vi "ExpandSearch.vi"(8 "error in (no error)":errorcluster, 11 "Waypoint in":refnum<class "Waypoint.lvclass">) -> (0 "error out":errorcluster, 2 "ExpandedSearchNodes":refnum<data-value>[](array[refnum]), 3 "Waypoint out":refnum<class "Waypoint.lvclass">)   [LabVIEW 2009, in "Waypoint.lvclass"]
uses:
  Waypoint.lvclass
  TreeNode/TreeNode.lvclass
  Waypoint.lvclass/Waypoint.ctl
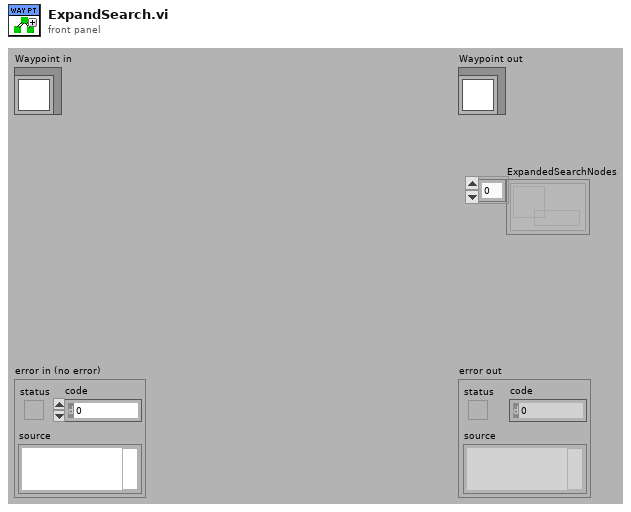
[diagram p1: front panel]
types:
  T1 = typedef "Waypoint.lvclass/point.ctl" = cluster{"X":dbl, "Y":dbl}
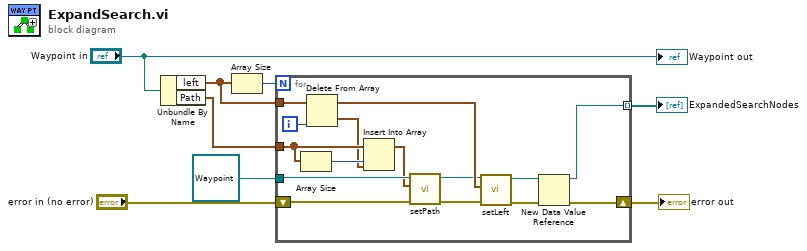
[diagram p0: block diagram]
diagram:
  n1 = Unbundle By Name("Waypoint in") -> ("left"=w7:T1[], "Path"=w1:T1[])
  n2 = Array Size(array=w7) -> (size(s)=w8:i32)
  n3 = for {
    N: w8 -> [_]
    tunnel: w7 -> [w23]
    tunnel: [w9] -> w5 mode=indexing
    shift-right: [w10] -> w3
    shift-left: "error in (no error)" -> [w14]
    tunnel: refnum<class "Waypoint.lvclass"> refnum ("Waypoint.lvclass") -> [w16]
    tunnel: w1 -> [w20]
    i -> [w22]
    n4 = Array Size(array=w20) -> (size(s)=w19:i32)
    n5 = Delete From Array(array=w23, index=w22) -> (deleted portion=w18:T1, array with subset deleted=w21:T1[])  [unwired: 1 in]
    n6 = Insert Into Array(array=w20, index=w19, new element=w18) -> (w15:T1[])
    n7 = call "setPath.vi"("error in (no error)"=w14, "Path"=w15, "Waypoint in"=w16) -> ("error out"=w13:errorcluster, "Waypoint out"=w17:refnum<class "Waypoint.lvclass">)  [unwired: 7 in]
    n8 = call "setLeft.vi"("error in (no error)"=w13, "left"=w21, "Waypoint in"=w17) -> ("error out"=w11:errorcluster, "Waypoint out"=w12:refnum<class "Waypoint.lvclass">)  [unwired: 7 in]
    n9 = New Data Value Reference(data value=w12, error in=w11) -> (data value reference=w9:refnum<data-value>, error out=w10:errorcluster)
  }
  "error out" <- w3
  "ExpandedSearchNodes" <- w5
  "Waypoint out" <- "Waypoint in"
